vi "Process PS Data.vi"(1 "PS Calibration":T2, 2 "Array":dbl[](array[numeric])) -> (0 "PS Indicator Cluster":T1 {"PS 6" scale=0.0..5.0 scale format="%#.2f"; "PS 5" scale=0.0..5.0 scale format="%#.2f"; "PS 4" scale=0.0..5.0 scale format="%#.2f"; "PS 3" scale=0.0..5.0 scale format="%#.2f"; "PS 2" scale=0.0..5.0 scale format="%#.2f"; "PS 1" scale=0.0..5.0 scale format="%#.2f"})   [LabVIEW 2017]
uses:
  Controls/PS Calibration Cluster.ctl
  Controls/PS Indicator Cluster.ctl
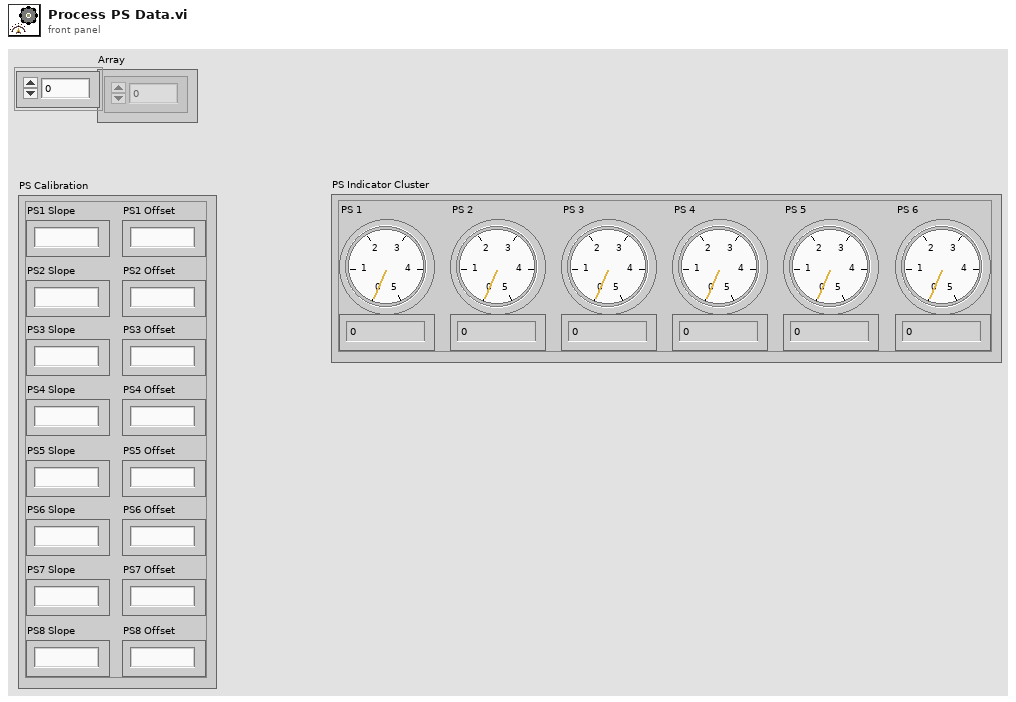
[diagram p1: front panel]
types:
  T1 = typedef "PS Indicator Cluster.ctl" = cluster{"PS 1":dbl, "PS 2":dbl, "PS 3":dbl, "PS 4":dbl, "PS 5":dbl, "PS 6":dbl}
  T2 = typedef "PS Calibration Cluster.ctl" = cluster{"PS1 Offset":string, "PS1 Slope":string, "PS2 Offset":string, "PS2 Slope":string, "PS3 Offset":string, "PS3 Slope":string, "PS4 Offset":string, "PS4 Slope":string, "PS5 Offset":string, "PS5 Slope":string, "PS6 Offset":string, "PS6 Slope":string, "PS7 Offset":string, "PS7 Slope":string, "PS8 Offset":string, "PS8 Slope":string}
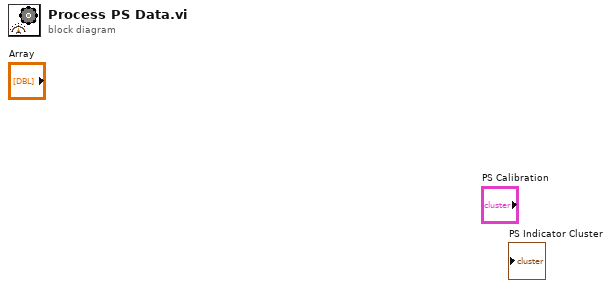
[diagram p0: block diagram]
diagram:
